vi "MainWerkendeOPGEKUISD.Vi"() -> ()   [LabVIEW 2013]
uses:
  <vilib>/Instr/_visa.llb/VISA Configure Serial Port (Instr).vi
panel:
  out "to hot":bool
  in  "vochtigheid graph to PNG file":path
  out "?":i32[](graph)
  in  "file path (use dialog)":path
  in  "setwaarde":string
  in  "themp graph to PNG file":path
  out "?":i32[](graph)
  in  "stop":bool
  out "vochtigheid":string
  out "temp":string
  in  "VISA resource name":refnum<visa-resource-name>
  # "in links out rechts (volgens de dataflow)"
  # "maakt gebruik van de NI visa driver . gelieven deze te dowloaden"
  # "als je de Vi afsluit moet je de arduino resetten(door op het knopje te drukken op het proto shield)"
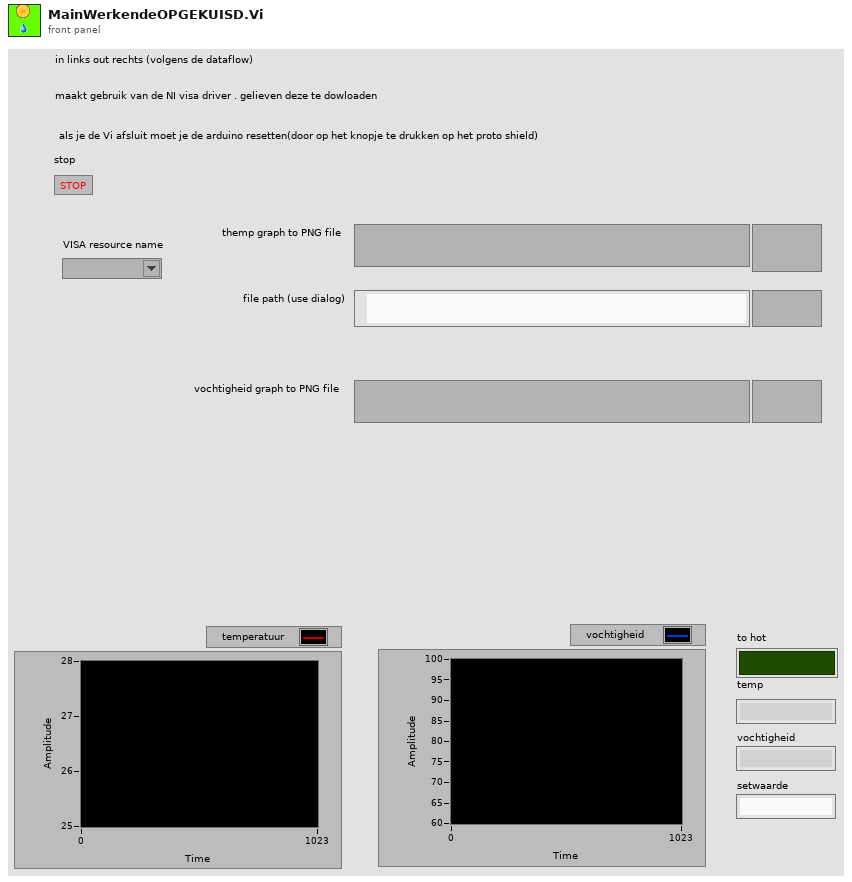
[diagram p1: front panel]
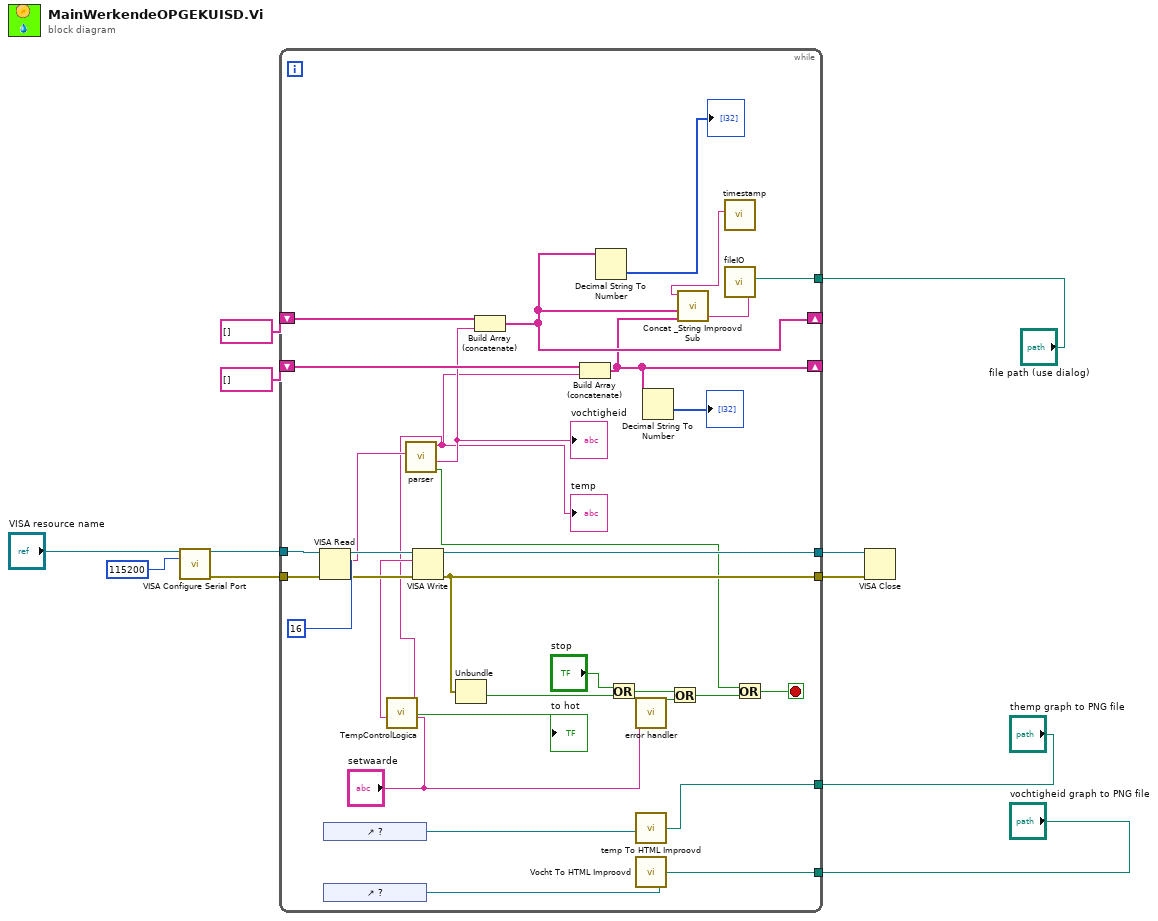
[diagram p0: block diagram]
diagram:
  n1 = call-poly "VISA Configure Serial Port"("VISA resource name"="VISA resource name", "baud rate (9600)"=u32 115200) -> ("VISA resource name out"=w11:refnum<visa-resource-name>, "error out"=w10:errorcluster)  [unwired: 12 in]
  n2 = while {
    tunnel: w11 -> [w44]
    tunnel: w10 -> [w43]
    tunnel: [w39] -> w7
    tunnel: [w38] -> w6
    shift-right: [w20] -> _
    shift-left: string[] [] -> [w37]
    shift-right: [w21] -> _
    shift-left: string[] [] -> [w36]
    tunnel: "vochtigheid graph to PNG file" -> [w18]
    tunnel: "file path (use dialog)" -> [w22]
    tunnel: "themp graph to PNG file" -> [w19]
    stop <- w30 stop-if-true
    n3 = VISA Read(VISA resource name=w44, byte count=u32 16, error in (no error)=w43) -> (VISA resource name out=w41:refnum<visa-resource-name>, read buffer=w16:string, error out=w40:errorcluster)  [unwired: 1 out]
    n4 = control-ref of="?"() -> (w17:refnum<vi>)
    n5 = control-ref of="?"() -> (w14:refnum<vi>)
    n6 = call "parser.vi"("input"=w16) -> ("temp"=w12:string, "vochtigheid"=w15:string, "error"=w13:bool)  [unwired: 7 in]
    "temp" <- w12
    "vochtigheid" <- w15
    n7 = call "TempControlLogica.vi"("setwaarde"="setwaarde", "input"=w12) -> ("output"=w24:string, "temp grooter dan setwaardde"=→"to hot":bool)  [unwired: 8 in]
    n8 = VISA Write(VISA resource name=w41, write buffer=w24, error in (no error)=w40) -> (VISA resource name out=w39:refnum<visa-resource-name>, error out=w38:errorcluster)  [unwired: 1 out]
    n9 = Unbundle(w38) -> ("status"=w33:bool)  [unwired: 2 out]
    n10 = Build Array (concatenate)(w36, w15) -> (w21:string[])
    n11 = Build Array (concatenate)(w37, w12) -> (w20:string[])
    n12 = Decimal String To Number(string=w21) -> (number=→"?":i32[])  [unwired: 2 in, 1 out]
    n13 = Or(x="stop", y=w33) -> (x .or. y?=w32:bool)
    n14 = call "error handler.vi"("setwaarde in"="setwaarde") -> ("Boolean"=w28:bool)  [unwired: 10 in]
    n15 = call "temp To HTML Improovd.vi"("temperatuur 3"=w17, "path to JPEG file"=w19) -> ()  [unwired: 4 in]
    n16 = call "Vocht To HTML Improovd.vi"("vochtigheid 4"=w14, "path to JPEG file"=w18) -> ()  [unwired: 4 in]
    n17 = Decimal String To Number(string=w20) -> (number=→"?":i32[])  [unwired: 2 in, 1 out]
    n18 = Or(x=w32, y=w28) -> (x .or. y?=w31:bool)
    n19 = call "timestamp.vi"() -> ("date/time string"=w27:string)  [unwired: 11 in]
    n20 = call "Concat _String Improovd Sub.vi"("vochtigheid"=w20, "temp"=w21, "timestamp"=w27) -> ("concat out"=w26:string)  [unwired: 8 in]
    n21 = call "fileIO.vi"("file path (use dialog)"=w22, "text"=w26) -> ()  [unwired: 8 in]
    n22 = Or(x=w13, y=w31) -> (x .or. y?=w30:bool)
  }
  n23 = VISA Close(VISA resource name=w7, error in (no error)=w6) -> ()  [unwired: 1 out]
